vi "Create.vi"(8 "error in (no error)":errorcluster, 9 "TCP":refnum<k5>, 10 "Request":refnum<class "Request.lvclass">) -> (0 "error out":errorcluster, 3 "WebSocket Client out":refnum<class "WebSocket Client.lvclass">)   [LabVIEW 2020, in "HTTP Server.lvlib" / "WebSocket Client.lvclass"]
uses:
  WebSocket Client.lvclass
  lv-http-util/HTTP Utils/Request/Request.lvclass
  Ref Data.ctl
  WebSocket Client.lvclass/WebSocket Client.ctl
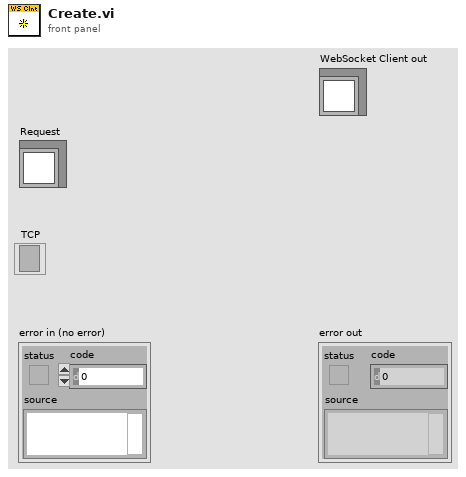
[diagram p1: front panel]
types:
  T1 = typedef "HTTP Server.lvlib/WebSocket Client.lvclass/Ref Data.ctl" = cluster{"Closing":bool}
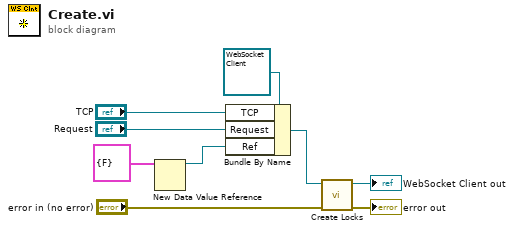
[diagram p0: block diagram]
diagram:
  n1 = New Data Value Reference(data value=T1 {"Closing"=FALSE} ("Ref Data")) -> (data value reference=w1:refnum<data-value>)  [unwired: 1 in, 1 out]
  n2 = Bundle By Name(cluster=refnum<class "WebSocket Client.lvclass"> refnum ("WebSocket Client in"), "TCP"="TCP", "Request"="Request", "Ref"=w1) -> (w4:refnum<class "WebSocket Client.lvclass">)
  n3 = call "Create Locks.vi"("error in (no error)"="error in (no error)", "WebSocket Client in"=w4) -> ("error out"=→"error out":errorcluster, "WebSocket Client out"=→"WebSocket Client out":refnum<class "WebSocket Client.lvclass">)  [unwired: 8 in]
